vi "restart.vi"(6 "Delay between send and receive [ms]":i32=100, 8 "error in (no error)":errorcluster, 11 "CCD in":refnum<class "CCD.lvclass">) -> (0 "error out":errorcluster, 1 "ID":i32, 2 "results-JSON string":string, 3 "CCD out":refnum<class "CCD.lvclass">)   [LabVIEW 2023, in "CCD.lvclass"]
doc: "Performs a restart on the CCD."
uses:
  CCD.lvclass
  CCD.lvclass/CCD.ctl
  20f7d3bd-08ac-4524-9bed-df36c1da25a0.vi
  GenericDevice/GenericDevice.lvclass
panel:
  # "Connector Pane"
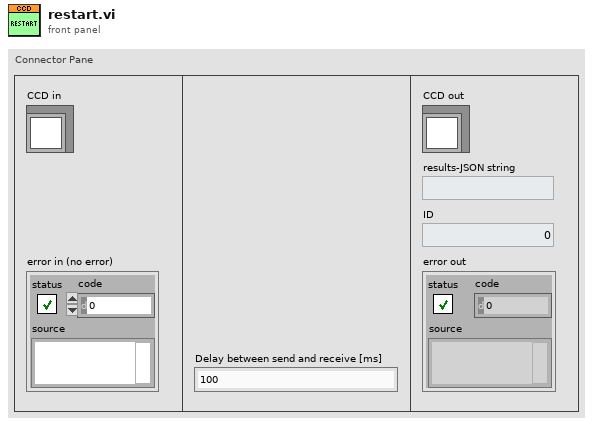
[diagram p1: front panel]
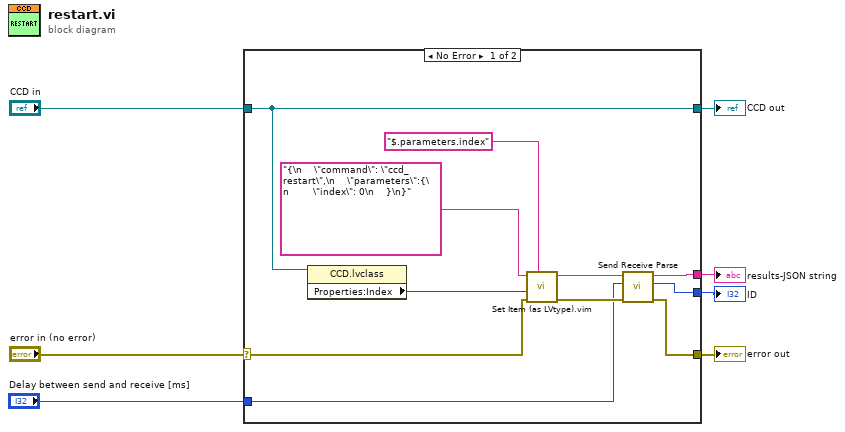
[diagram p0: block diagram]
diagram:
  n1 = case shown="No Error" "error in (no error)" {
    selector: "error in (no error)" -> [w14 w20]
    tunnel: [w13 w20] -> w6
    tunnel: [w16 w19] -> w4
    tunnel: "CCD in" -> [w16 w19]
    tunnel: [w12 _] -> w3
    tunnel: [w11 _] -> w2
    tunnel: "Delay between send and receive [ms]" -> [w9 _]
    frame No Error {
      n2 = property class="CCD.lvclass"(reference=w16) -> ("Properties:Index"=w15:i32)  [unwired: 1 in, 2 out]
      n3 = call "Set Item (as LVtype).vim"("$Path or Item Name"="$.parameters.index", "error in (no error)"=w14, "Anything"=w15, "JSON"="{\n    \"command\": \"ccd_restart\",\n    \"parameters\":{\n        \"index\": 0\n    }\n}") -> ("error out"=w10:errorcluster, "<JSON>"=w8:string)  [unwired: 4 in, 1 out]
      n4 = call "Send Receive Parse.vi"("error in"=w10, "Delay between send and receive [ms]"=w9, "<JSON>"=w8) -> ("error out"=w13:errorcluster, "ID"=w11:i32, "results-JSON string"=w12:string)  [unwired: 6 in]
    }
    frame Error {
    }
  }
  "error out" <- w6
  "CCD out" <- w4
  "results-JSON string" <- w3
  "ID" <- w2
